vi "Configure Data Save.vi"(0 "VISA resource name":refnum<visa-resource-name>, 1 "Data File Name Identified Strings (\"\")":string, 2 "Media Auto Save (On)":bool=TRUE, 3 "Media FIFO (Off)":bool, 5 "Save Directory Name (\"DATA0\")":string="DATA0", 7 "File Header Characters (\"\")":string, 9 "Data File Name Structure (0: Date)":u16(ring) items=["Date", "Serial", "Batch"], 11 "error in (no error)":errorcluster, 12 "File Format (0: Binary)":u16(ring) items=["Binary", "Text"]) -> (4 "VISA resource name out":refnum<visa-resource-name>, 15 "error out":errorcluster)   [LabVIEW 2020, in "Yokogawa GX Series.lvlib"]
doc: "Sets the configuation of saving data.\n\nCommands: SDirectory, SFileHead, SFileName, SMediaSave, SFileFormat"
uses:
  <instrlib>/Yokogawa GX Series/Yokogawa GX Series.lvlib
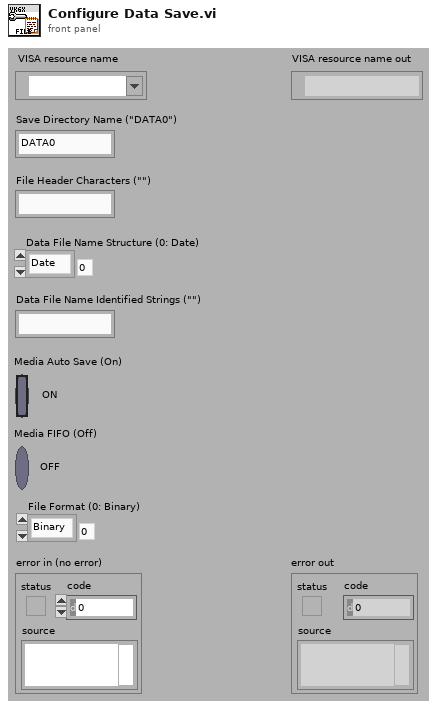
[diagram p1: front panel]
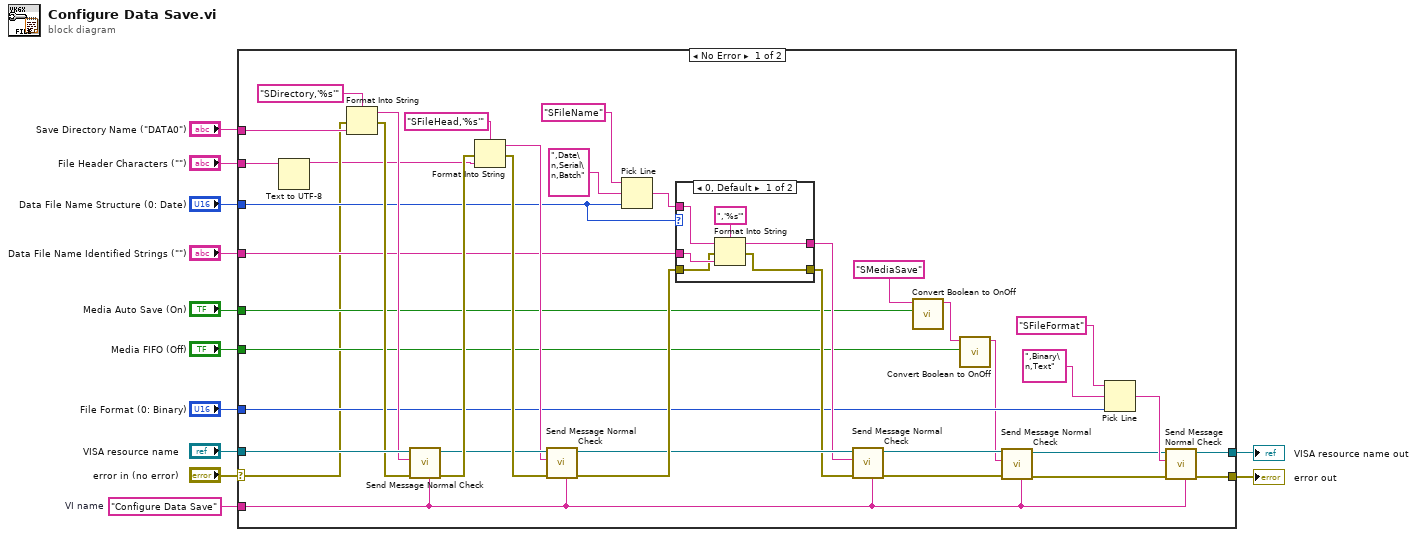
[diagram p0: block diagram]
diagram:
  w4 = "Configure Data Save"  # VI name
  n1 = case shown="No Error" "error in (no error)" {
    selector: "error in (no error)" -> [w16 w59]
    tunnel: "VISA resource name" -> [w50 w60]
    tunnel: "Save Directory Name (\"DATA0\")" -> [w48 _]
    tunnel: "File Header Characters (\"\")" -> [w14 _]
    tunnel: "Data File Name Structure (0: Date)" -> [w39 _]
    tunnel: "Data File Name Identified Strings (\"\")" -> [w37 _]
    tunnel: "File Format (0: Binary)" -> [w28 _]
    tunnel: [w24 w60] -> w6
    tunnel: [w23 w59] -> w5
    tunnel: w4 -> [w22 _]
    tunnel: "Media Auto Save (On)" -> [w21 _]
    tunnel: "Media FIFO (Off)" -> [w18 _]
    frame No Error {
      n2 = Text to UTF-8(11:w14) -> (3:w13:string)  [unwired: 2 in, 1 out]
      n3 = Format Into String(format string="SDirectory,'%s'", error in=w16, w48) -> (resulting string=w46:string, error out=w47:errorcluster)  [unwired: 1 in]
      n4 = call <instrlib>:"Send Message Normal Check.vi"("Source (\"\")"=w22, "error in (no error)"=w47, "Send Message (\"\")"=w46, "VISA resource name"=w50) -> ("error out"=w44:errorcluster, "VISA resource name out"=w42:refnum<visa-resource-name>)  [unwired: 2 in, 4 out]
      n5 = Format Into String(format string="SFileHead,'%s'", error in=w44, w13) -> (resulting string=w41:string, error out=w43:errorcluster)  [unwired: 1 in]
      n6 = call <instrlib>:"Send Message Normal Check.vi"("Source (\"\")"=w22, "error in (no error)"=w43, "Send Message (\"\")"=w41, "VISA resource name"=w42) -> ("error out"=w36:errorcluster, "VISA resource name out"=w35:refnum<visa-resource-name>)  [unwired: 2 in, 4 out]
      n7 = Pick Line(string ("")="SFileName", multi-line string=",Date\n,Serial\n,Batch", line index=w39) -> (output string=w38:string)
      n8 = case shown="0, Default" w39 {
        tunnel: w38 -> [w56 w58]
        tunnel: w37 -> [w54 _]
        tunnel: w36 -> [w53 w57]
        tunnel: [w52 w57] -> w34
        tunnel: [w51 w58] -> w33
        frame 0, Default {
          n9 = Format Into String(format string=",'%s'", initial string=w56, error in=w53, w54) -> (resulting string=w51:string, error out=w52:errorcluster)
        }
        frame 2 {
        }
      }
      n10 = call <instrlib>:"Send Message Normal Check.vi"("Source (\"\")"=w22, "error in (no error)"=w34, "Send Message (\"\")"=w33, "VISA resource name"=w35) -> ("error out"=w31:errorcluster, "VISA resource name out"=w32:refnum<visa-resource-name>)  [unwired: 2 in, 4 out]
      n11 = call <instrlib>:"Convert Boolean to OnOff.vi"("On/Off"=w21, "Initial String (\"\")"="SMediaSave") -> ("Resulting String"=w19:string)  [unwired: 9 in]
      n12 = call <instrlib>:"Convert Boolean to OnOff.vi"("On/Off"=w18, "Initial String (\"\")"=w19) -> ("Resulting String"=w17:string)  [unwired: 9 in]
      n13 = call <instrlib>:"Send Message Normal Check.vi"("Source (\"\")"=w22, "error in (no error)"=w31, "Send Message (\"\")"=w17, "VISA resource name"=w32) -> ("error out"=w25:errorcluster, "VISA resource name out"=w26:refnum<visa-resource-name>)  [unwired: 2 in, 4 out]
      n14 = Pick Line(string ("")="SFileFormat", multi-line string=",Binary\n,Text", line index=w28) -> (output string=w27:string)
      n15 = call <instrlib>:"Send Message Normal Check.vi"("Source (\"\")"=w22, "error in (no error)"=w25, "Send Message (\"\")"=w27, "VISA resource name"=w26) -> ("error out"=w23:errorcluster, "VISA resource name out"=w24:refnum<visa-resource-name>)  [unwired: 2 in, 4 out]
    }
    frame Error {
    }
  }
  "error out" <- w5
  "VISA resource name out" <- w6
